vi "Get Events.vi"(11 "Test Node View in":refnum<class "Test Node View.lvclass">) -> (2 "Events":T1, 3 "Test Node View out":refnum<class "Test Node View.lvclass">)   [LabVIEW 2013, in "Test Node View.lvlib" / "Test Node View.lvclass"]
uses:
  Test Node View.lvclass
  Typedef/Events.ctl
  Test Node View.lvclass/Test Node View.ctl
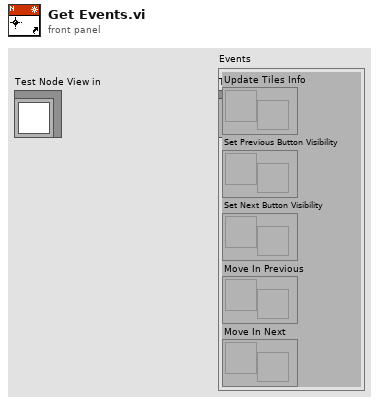
[diagram p1: front panel]
types:
  T1 = typedef "Test Node View.lvlib/Test Node View.lvclass/Events.ctl" = cluster{"Update Tiles Info":refnum<user-event>, "Set Previous Button Visibility":refnum<user-event>, "Set Next Button Visibility":refnum<user-event>, "Move In Previous":refnum<user-event>, "Move In Next":refnum<user-event>}
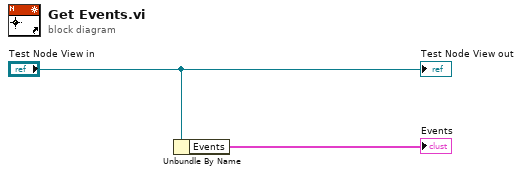
[diagram p0: block diagram]
diagram:
  n1 = Unbundle By Name("Test Node View in") -> ("Events"=→"Events":T1)
  "Test Node View out" <- "Test Node View in"
